vi "Log_String.vi"(10 "Message":string, 11 "EventLog":refnum<class "abs_EventLog.lvclass">) -> (3 "node out":refnum<class "bt_Log.lvclass">)   [LabVIEW 2021, in "BT.lvlib"]
uses:
  BT.lvlib
  Nodes/Leaves/Log/bt_Log.lvclass
  <vilib>/TSA/Event Log/abs_EventLog/abs_EventLog.lvclass
  <vilib>/TSA/Abstract Data Classes/Constants/Support/Str/Str.vi
  <vilib>/TSA/Abstract Data Classes/Constants/Support/Str/Const_Str.lvclass
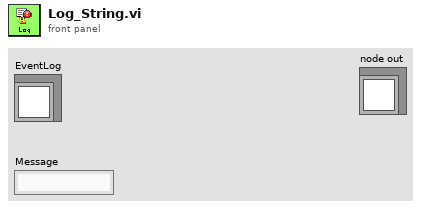
[diagram p1: front panel]
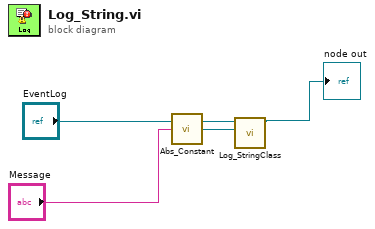
[diagram p0: block diagram]
diagram:
  n1 = call-poly <vilib>:"Abs_Constant.vi"("String"="Message") -> ("Abs_String.lvclass"=w1:refnum<class "Abs_String.lvclass">)  [unwired: 4 in]
  n2 = call "Log_StringClass.vi"("Message"=w1, "EventLog"="EventLog") -> ("node out"=→"node out":refnum<class "bt_Log.lvclass">)  [unwired: 9 in]
